vi "SubVI_CalculateRange.vi"(8 "XScale.Minimum":dbl, 9 "XScale.Maximum":dbl, 10 "File End Time":dbl, 11 "File Start Time":dbl) -> (3 "Range":cluster{dbl, dbl})   [LabVIEW 2012]
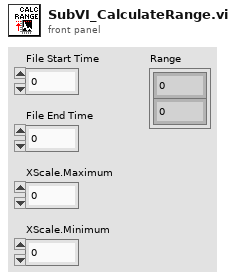
[diagram p1: front panel]
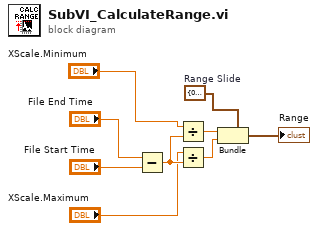
[diagram p0: block diagram]
diagram:
  w8 = cluster{dbl, dbl} {0.44603381014304294, 0.5370611183355006}  # Range Slide
  n1 = Subtract(x="File End Time", y="File Start Time") -> (x-y=w2:dbl)
  n2 = Divide(x="XScale.Minimum", y=w2) -> (x/y=w7:dbl)
  n3 = Divide(x="XScale.Maximum", y=w2) -> (x/y=w6:dbl)
  n4 = Bundle(cluster=w8, w7, w6) -> (→"Range":cluster{dbl, dbl})
